vi "EOLCheck.vi"(11 "Console":string) -> (3 "waiting....":bool)   [LabVIEW 2021]
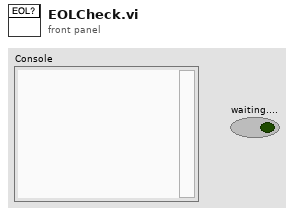
[diagram p1: front panel]
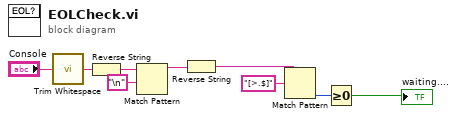
[diagram p0: block diagram]
diagram:
  n1 = call <vilib>:"Trim Whitespace.vi"("string"="Console") -> ("trimmed string"=w1:string)  [unwired: 1 in]
  n2 = Reverse String(1:w1) -> (0:w8:string)
  n3 = Match Pattern(string=w8, regular expression="\n") -> (before substring=w6:string)  [unwired: 1 in, 3 out]
  n4 = Reverse String(1:w6) -> (0:w5:string)
  n5 = Match Pattern(string=w5, regular expression="[>.$]") -> (offset past match=w3:i32)  [unwired: 1 in, 3 out]
  n6 = Greater Or Equal To 0?(x=w3) -> (x >= 0?=→"waiting....":bool)
